vi "RD Digital Uart Rx.vi"(0 "handle":u64, 7 "length":i32, 11 "error in (no error)":errorcluster caption="错误输入（无错误）") -> (3 "fParity out":i32, 4 "handle out":u64, 6 "rgRX":u8[](array[numeric]), 8 "function return":i32, 10 "rxcount out":i32, 15 "error out":errorcluster caption="错误输出")   [LabVIEW 2018, in "InstrumentsPlayground.lvlib"]
doc: "CLIFFAPI int CliffDigitalUartRx(FT_HANDLE handle, uchar* rgRX, int length, int * rxcount, int *fParity);"
uses:
  InstrumentsPlayground.lvlib
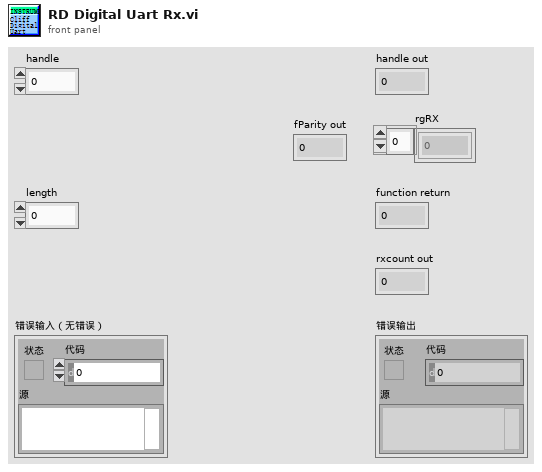
[diagram p1: front panel]
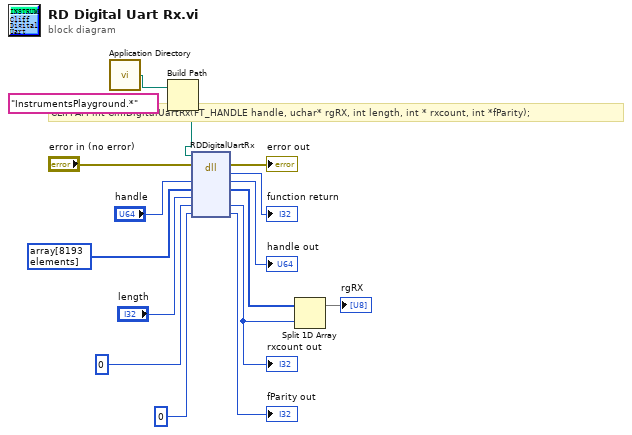
[diagram p0: block diagram]
diagram:
  # "CLIFFAPI int CliffDigitalUartRx(FT_HANDLE handle, uchar* rgRX, int length, int * rxcount, int *fParity);"
  n1 = call <vilib>:"Application Directory.vi"() -> ("Application Directory"=w6:path)
  n2 = Build Path(base path=w6, name or relative path="InstrumentsPlayground.*" ("名称或相对路径")) -> (appended path=w5:path)
  n3 = dll-call lib="E:/work/YZCourse_Xtext/Cliff/API/LabVIEW lib/InstrumentsPlayground.*" fn="RDDigitalUartRx"(path in=w5, error in="error in (no error)", "handle"="handle", "rgRX"=u8[] array[8193 elements], "length"="length", "rxcount"=0, "fParity"=0) -> (error out=→"error out":errorcluster, "返回类型"=→"function return":i32, "handle"=→"handle out":u64, "rgRX"=w4:u8[], "rxcount"=w2:i32, "fParity"=→"fParity out":i32)  [unwired: 2 in, 1 out]
  "rxcount out" <- w2
  n4 = Split 1D Array(array=w4, index=w2) -> (first subarray=→"rgRX":u8[])  [unwired: 1 out]
